vi "Get_LabVIEW_default_printer_name.vi"(1 "error in (no error)":errorcluster) -> (3 "Get Default Printer":string, 4 "error out":errorcluster)   [LabVIEW 2017, in "NI_ReportGenerationCore.lvlib"]
uses:
  <vilib>/Utility/NIReport.llb/NI_ReportGenerationCore.lvlib
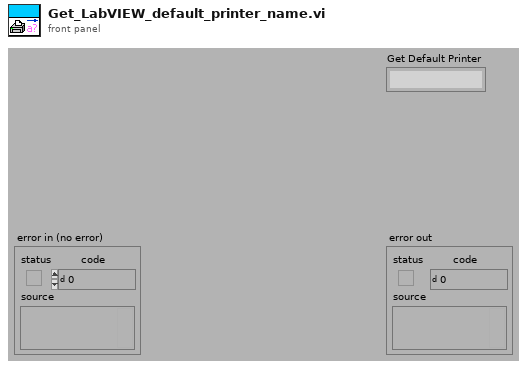
[diagram p1: front panel]
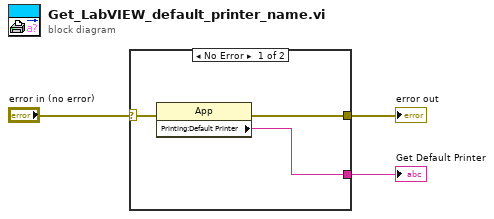
[diagram p0: block diagram]
diagram:
  n1 = case shown="No Error" "error in (no error)" {
    selector: "error in (no error)" -> [w5 w7]
    tunnel: [w6 w7] -> w3
    tunnel: [w4 _] -> w1
    frame No Error {
      n2 = property class="App"(error in=w5) -> (error out=w6:errorcluster, "Printing:Default Printer"=w4:string)  [unwired: 1 in, 1 out]
    }
    frame Error {
    }
  }
  "error out" <- w3
  "Get Default Printer" <- w1
